vi "testBlockDMA_GERM.vi"(8 "error in (no error)":errorcluster, 11 "TestCase in":refnum<class "DSF CD System Tests.lvclass">) -> (0 "error out":errorcluster, 3 "TestCase out":refnum<class "DSF CD System Tests.lvclass">)   [LabVIEW 2017, in "DSF CD System Tests.lvclass"]
uses:
  DSF CD System Tests.lvclass
  C:/Git/niveristand-custom-device-testing-tools/VeriStandTestCase/VeriStandTestCase.lvclass
  <vilib>/NI/GE Reflective Memory Driver/Typedefs/GE 5565PIORC.Typedef.DMA Wait Mode.ctl
  fe7e187c-5126-4982-8e63-bd07b26320cd.vi
  <vilib>/NI/GE Reflective Memory Driver/GE 5565PIORC.lvclass
  <vilib>/addons/_JKI Toolkits/VI Tester/TestCase.llb/TestCase.lvclass
  C:/Program Files (x86)/National Instruments/LabVIEW 2017/vi.lib/addons/_JKI Toolkits/VI Tester/TestCase.llb/TestCase.lvclass
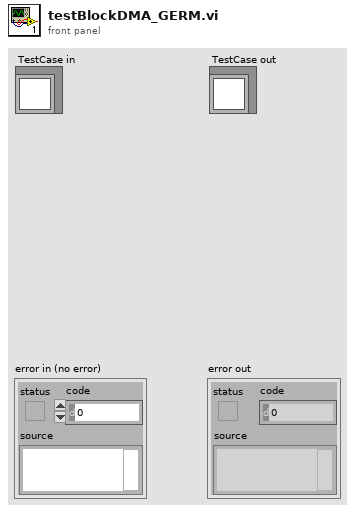
[diagram p1: front panel]
types:
  T1 = typedef "GE 5565PIORC.lvclass/GE 5565PIORC.Typedef.DMA Wait Mode.ctl" = enum16{"Polling", "Interrupt"}
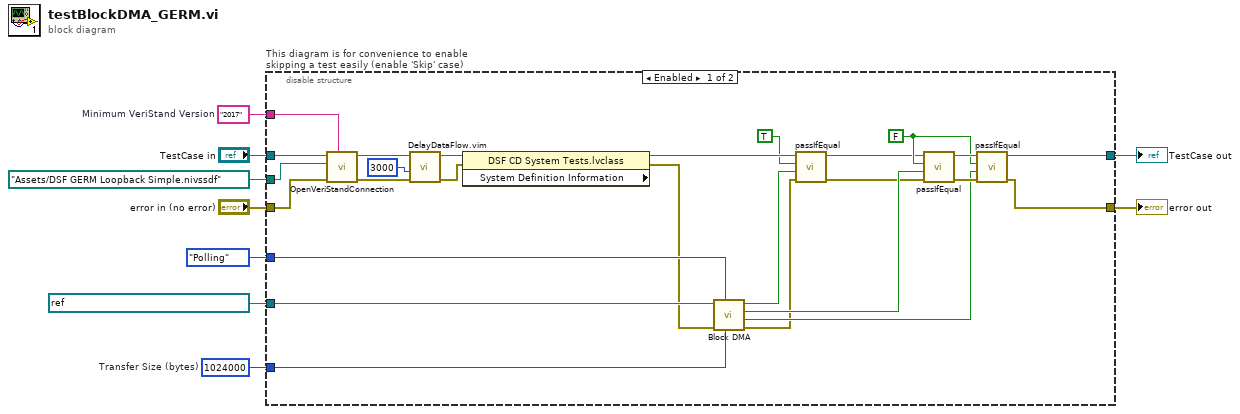
[diagram p0: block diagram]
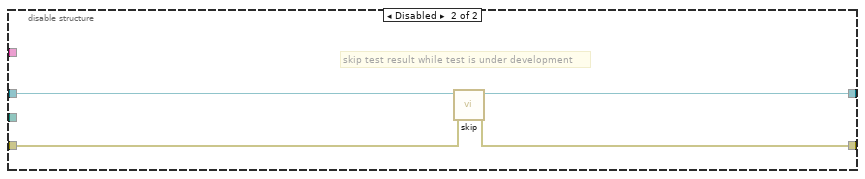
[diagram p2: hidden frame]
diagram:
  w2 = u32 1024000  # Transfer Size (bytes)
  w4 = "2017"  # Minimum VeriStand Version
  n1 = disable-structure "This diagram is for convenience to enable skipping a test easily (enable 'Skip' case)" shown="Enabled" {
    disable-tunnel: "TestCase in" -> [w34 w38]
    disable-tunnel: [w30 w36] -> w8
    disable-tunnel: [w28 w37] -> w7
    disable-tunnel: "error in (no error)" -> [w26 w35]
    disable-tunnel: path "Assets/DSF GERM Loopback Simple.nivssdf" ("System Definition File") -> [w33 _]
    disable-tunnel: w4 -> [w32 _]
    disable-tunnel: GE_5565PIORC.Typedef.DMA_Wait_Mode."Polling" ("Wait Mode") -> [w25 _]
    disable-tunnel: w2 -> [w22 _]
    disable-tunnel: refnum<visa-resource-name> "visa://10.2.109.77/PXI8::15::INSTR" ("VISA Resource Name") -> [w24 _]
    frame Enabled {
      w27 = FALSE ("timed out?")
      n2 = call-dynamic "OpenVeriStandConnection.vi"("Minimum VeriStand Version (2016)"=w32, "error in (no error)"=w26, "System Definition File"=w33, "VeriStand Test Case in"=w34) -> ("error out"=w11:errorcluster, "VeriStand Test Case out"=w13:refnum<class "DSF CD System Tests.lvclass">)  [unwired: 5 in, 1 out]
      n3 = call "DelayDataFlow.vim"("value in"=w11, "milliseconds to wait"=u32 3000) -> ("value out"=w10:errorcluster)  [unwired: 2 in, 1 out]
      n4 = property class="DSF CD System Tests.lvclass" props=["System Definition Information"](reference=w13, error in=w10) -> (reference out=w20:refnum<class "DSF CD System Tests.lvclass">, error out=w23:errorcluster)  [unwired: 1 out]
      n5 = call "Block DMA.vi"("Transfer Size (bytes)"=w22, "Wait Mode"=w25, "error in (no error)"=w23, "VISA Resource Name"=w24) -> ("error out"=w15:errorcluster, "Read Timed Out?"=w16:bool, "Write Timed Out?"=w21:bool, "Success?"=w17:bool)  [unwired: 4 in]
      n6 = call-dynamic "passIfEqual.vi"("error in (no error)"=w15, "y"=w17, "x"=TRUE ("timed out?"), "TestCase in"=w20) -> ("error out"=w14:errorcluster, "TestCase out"=w19:refnum<class "DSF CD System Tests.lvclass">)  [unwired: 6 in]
      n7 = call-dynamic "passIfEqual.vi"("error in (no error)"=w14, "y"=w21, "x"=w27, "TestCase in"=w19) -> ("error out"=w29:errorcluster, "TestCase out"=w31:refnum<class "DSF CD System Tests.lvclass">)  [unwired: 6 in]
      n8 = call-dynamic "passIfEqual.vi"("error in (no error)"=w29, "y"=w16, "x"=w27, "TestCase in"=w31) -> ("error out"=w28:errorcluster, "TestCase out"=w30:refnum<class "DSF CD System Tests.lvclass">)  [unwired: 6 in]
    }
    frame Disabled {
      # "skip test result while test is under development"
      n9 = call <vilib>:"skip.vi"("error in (no error)"=w35, "TestCase in"=w38) -> ("error out"=w37:errorcluster, "TestCase out"=w36:refnum<class "DSF CD System Tests.lvclass">)  [unwired: 8 in]
    }
  }
  "error out" <- w7
  "TestCase out" <- w8
